vi "array of strings json test.vi"() -> ()   [LabVIEW 2013]
uses:
  JSONtext.lvlib
panel:
  out "labview's bad version":cluster{"subs":string[]}[](array[cluster])
  out "labview mishandles null":bool
  out "<JSON>":string
  out "unflattened correctly":cluster{"subs":string[]}[](array[cluster])
  out "error out":errorcluster
  out "jsontext ok":bool
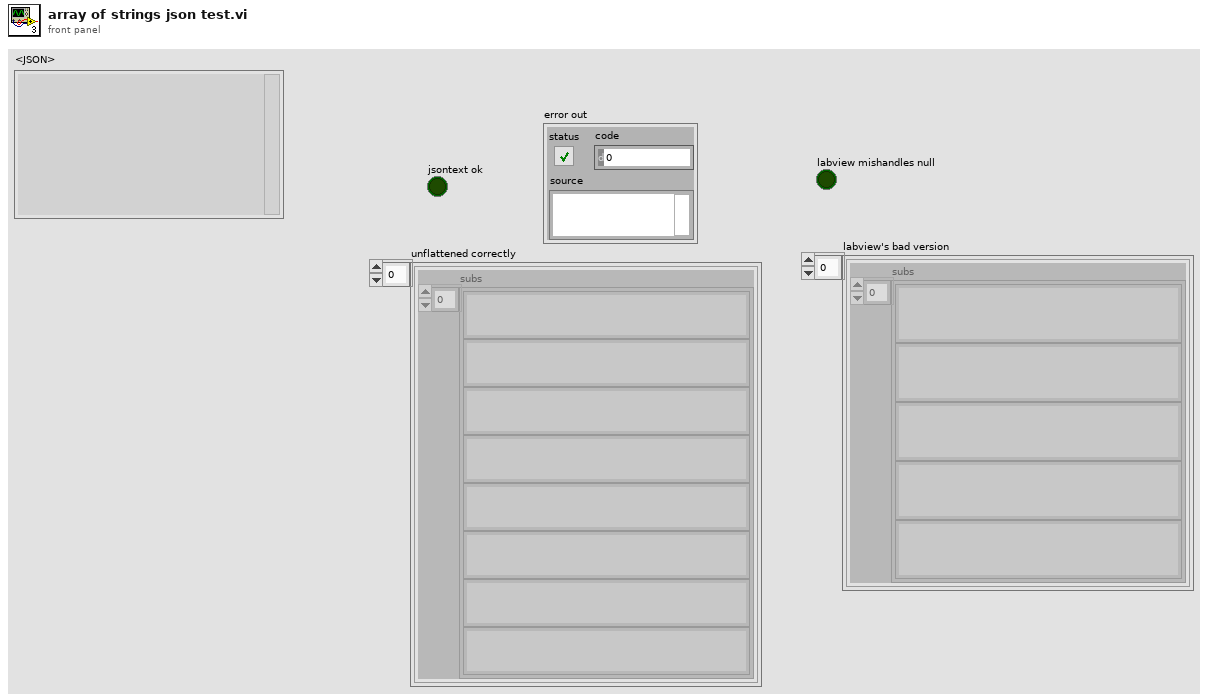
[diagram p1: front panel]
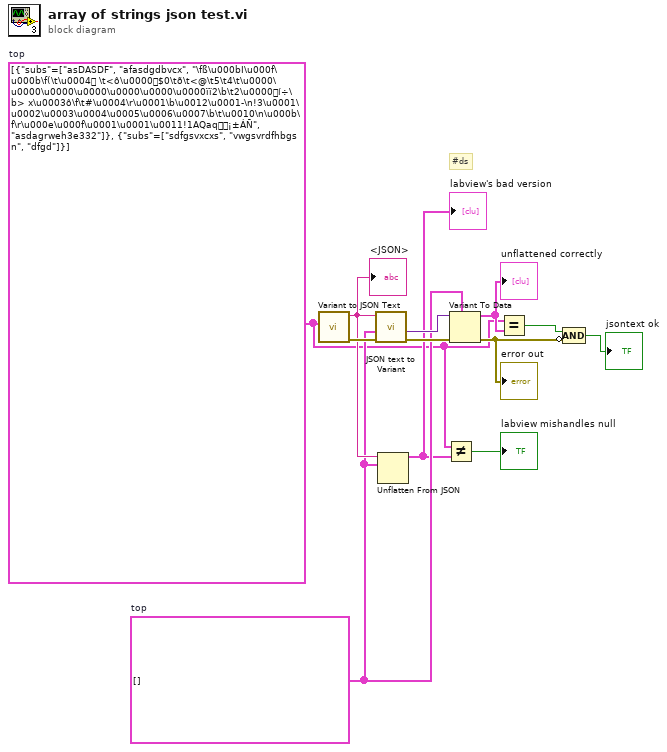
[diagram p0: block diagram]
diagram:
  w2 = cluster{"subs":string[]}[] [{"subs"=["asDASDF", "afasdgdbvcx", "\fß\u000bI\u000f\u000b\f(\t\u0004 \t<ô\u0000$0\tð\t<@\t5\t4\t\u0000\u0000\u0000\u0000\u0000\u0000\u0000ïï2\b\t2\u0000í÷\b> x\u0003ô\f\t#\u0004\r\u0001\b\u0012\u0001-\n!3\u0001\u0002\u0003\u0004\u0005\u0006\u0007\b\t\u0010\n\u000b\f\r\u000e\u000f\u0001\u0001\u0011!1AQaq¡±ÁÑ", "asdagrweh3e332"]}, {"subs"=["sdfgsvxcxs", "vwgsvrdfhbgs n", "dfgd"]}]  # top
  w4 = cluster{"subs":string[]}[] []  # top
  # "#ds"
  n1 = call "Variant to JSON Text.vi"("Variant"=w2) -> ("error out"=w10:errorcluster, "<JSON>"=w5:string)  [unwired: 9 in]
  "<JSON>" <- w5
  n2 = call "JSON text to Variant.vi"("error in (no error)"=w10, "Data Type"=w4, "JSON"=w5) -> ("error out"=w11:errorcluster, "Variant out"=w12:variant)  [unwired: 7 in]
  n3 = Unflatten From JSON(JSON string=w5, type and defaults=w4) -> (value=w3:cluster{"subs":string[]}[])  [unwired: 5 in, 1 out]
  "labview's bad version" <- w3
  n4 = Not Equal?(x=w2, y=w3) -> (x != y?=→"labview mishandles null":bool)
  n5 = Variant To Data(error in=w11, type=w4, Variant=w12) -> (data=w6:cluster{"subs":string[]}[], error out=w8:errorcluster)
  "error out" <- w8
  "unflattened correctly" <- w6
  n6 = Equal?(x=w2, y=w6) -> (x = y?=w9:bool)
  n7 = Compound Arithmetic op=AND(w9, invert w8) -> (→"jsontext ok":bool)
